vi "QuerryCustomUserCommand.vi"(7 "Mode":enum16{"Set", "GetAndRemove", "DeleteAll"}(ring), 8 "error in (no error)":errorcluster, 10 "STR_UserCommand":string, 11 "VISA Refnum in":refnum<visa-resource-name>) -> (0 "error out":errorcluster, 3 "communication_data":T1)   [LabVIEW 2018]
uses:
  OXYGEN/TypeDefs/Cluster_RawCommData.ctl
  OXYGEN.lvlib
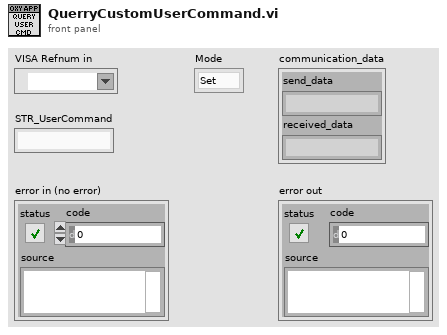
[diagram p1: front panel]
types:
  T1 = typedef "OXYGEN.lvlib/Cluster_RawCommData.ctl" = cluster{"send_data":string, "received_data":string}
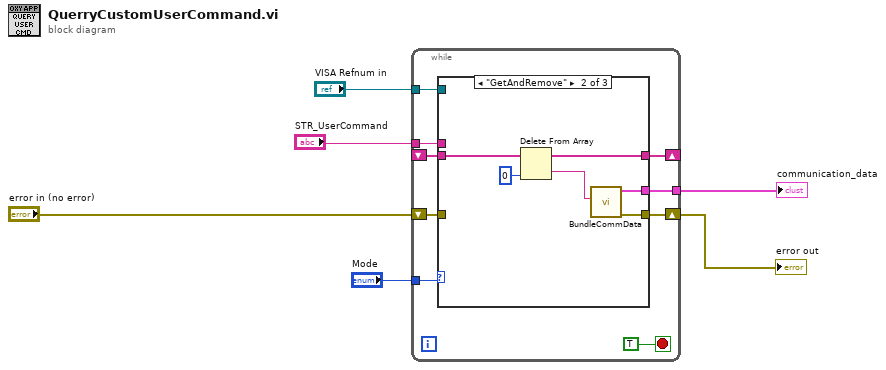
[diagram p0: block diagram]
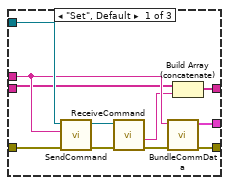
[diagram p2: hidden frame]
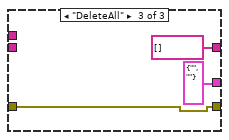
[diagram p3: hidden frame]
diagram:
  n1 = while {
    tunnel: "STR_UserCommand" -> [w15]
    tunnel: [w14] -> w5
    tunnel: "VISA Refnum in" -> [w12]
    shift-right: [w13] -> w4
    shift-left: "error in (no error)" -> [w11]
    tunnel: "Mode" -> [w10]
    shift-right: [w9] -> _
    shift-left: _ -> [w7]
    stop <- TRUE stop-if-true
    n2 = case shown="\"GetAndRemove\"" w10 {
      tunnel: w15 -> [w20 _ _]
      tunnel: [w19 w32 T1 {"send_data"="", "received_data"=""} ("communication_data")] -> w14
      tunnel: [w22 w31 w33] -> w13
      tunnel: w12 -> [w26 _ _]
      tunnel: w11 -> [w24 _ w33]
      tunnel: [w17 w29 string[] []] -> w9
      tunnel: w7 -> [w18 w30 _]
      frame "Set", Default {
        n3 = call "SendCommand.vi"("error in (no error)"=w24, "String to Send"=w20, "OXY_SCPI Reseource In"=w26) -> ("error out"=w21:errorcluster, "OXY_SCPI Reseource Out"=w25:refnum<visa-resource-name>)  [unwired: 7 in]
        n4 = call "ReceiveCommand.vi"("error in (no error)"=w21, "OXY_SCPI Reseource In"=w25) -> ("error out"=w23:errorcluster, "received Data with Header"=w16:string)  [unwired: 6 in, 2 out]
        n5 = call "BundleCommData.vi"("error in (no error)"=w23, "send_data"=w20) -> ("error out"=w22:errorcluster, "communication_data"=w19:T1)  [unwired: 8 in]
        n6 = Build Array (concatenate)(w18, w16) -> (w17:string[])
      }
      frame "GetAndRemove" {
        n7 = Delete From Array(array=w30, index=0) -> (deleted portion=w28:string, array with subset deleted=w29:string[])  [unwired: 1 in]
        n8 = call "BundleCommData.vi"("received_data"=w28) -> ("error out"=w31:errorcluster, "communication_data"=w32:T1)  [unwired: 9 in]
      }
      frame "DeleteAll" {
      }
    }
  }
  "communication_data" <- w5
  "error out" <- w4
